vi "(C2K_ADC)_Config_Sweeps.vi"(8 "Error In":errorcluster, 10 "Parameter":T2, 11 "Front Panel Pop up":bool=TRUE) -> (0 "Error Out":errorcluster, 1 "VDDA":dbl[](array[numeric]), 2 "VDD":dbl[](array[numeric]), 3 "Temp":dbl[](array[numeric]), 4 "Parameter Out":T2, 5 "VDDIO":dbl[](array[numeric]))   [LabVIEW 2019]
uses:
  (C2K_ADC)_Array_cell_En_Dis.ctl
  (C2K_ADC)_Parameter.ctl
  (C2K_ADC)_Global.vi
panel:
  in  "VDDIO":T1
  out "name":string
  in  "Cancel Button":bool
  in  "OK Button":bool
  in  "Load Config":bool
  in  "Save Config":bool
  in  "VDDA":T1
  in  "VDD":T1
  in  "Temp":T1
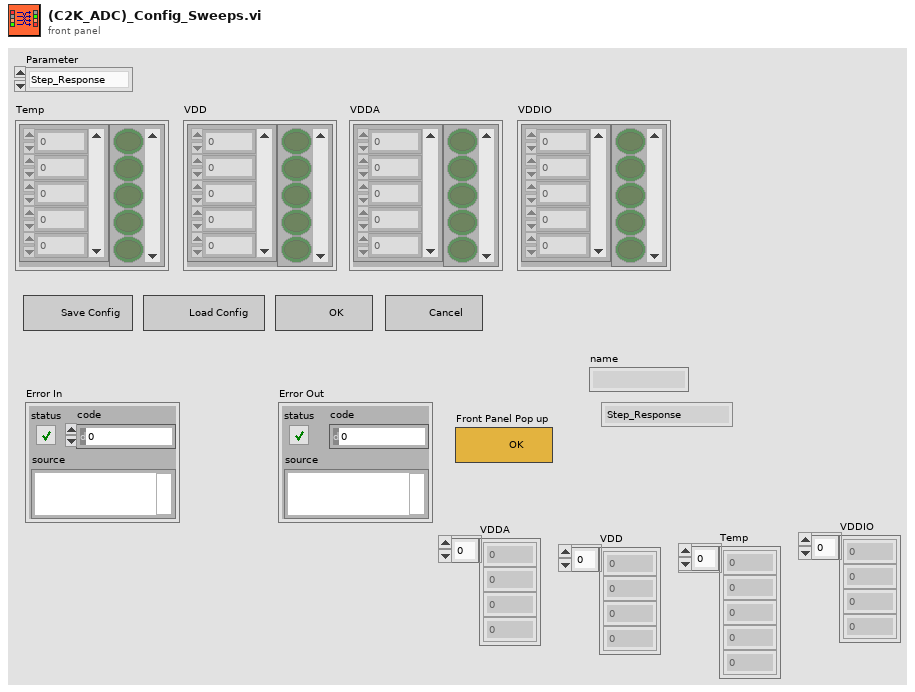
[diagram p1: front panel]
types:
  T1 = typedef "(C2K_ADC)_Array_cell_En_Dis.ctl" = cluster{"Array":dbl[], "Array 3":bool[]}
  T2 = typedef "(C2K_ADC)_Parameter.ctl" = enum16{"Step_Response"}
  T3 = enum32{"Invalid", "Standard", "Closed", "Hidden", "Minimized", "Maximized"}
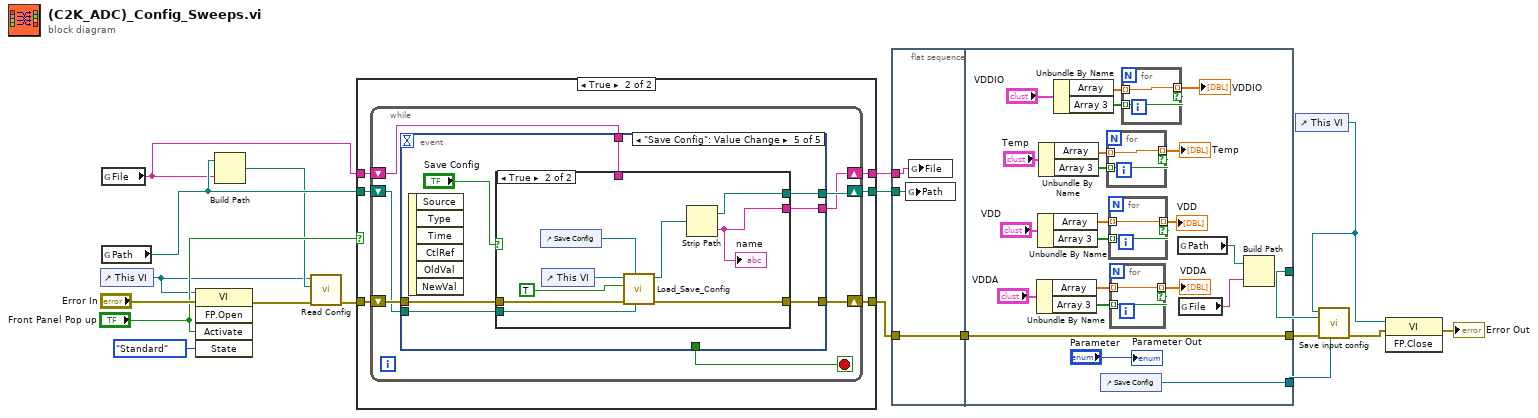
[diagram p0: block diagram]
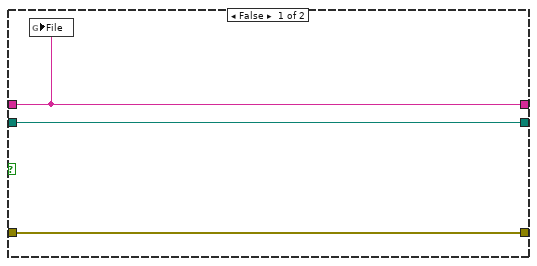
[diagram p2: hidden frame]
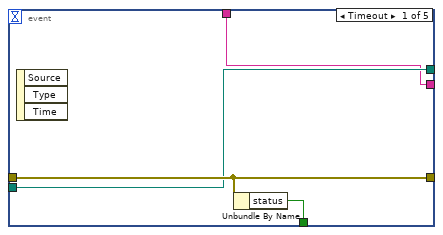
[diagram p3: hidden frame]
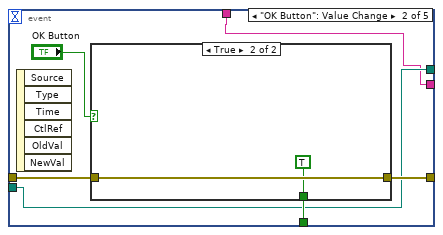
[diagram p4: hidden frame]
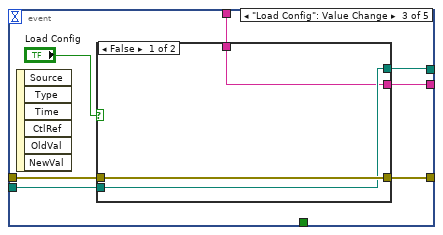
[diagram p6: hidden frame]
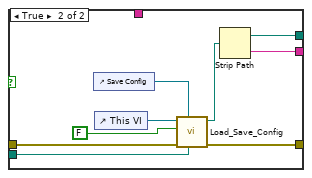
[diagram p7: hidden frame]
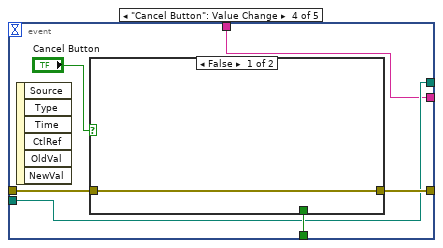
[diagram p8: hidden frame]
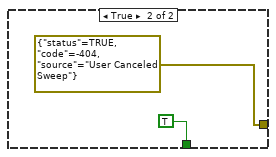
[diagram p9: hidden frame]
diagram:
  n1 = control-ref of="This VI"() -> (w9:refnum<vi>)
  n2 = global read "(C2K_ADC)_Global.vi" "File"() -> (w8:string)
  n3 = global read "(C2K_ADC)_Global.vi" "Path"() -> (w14:path)
  n4 = invoke class="VI" method="FP.Open"(reference=w9, error in="Error In", "Activate"="Front Panel Pop up", "State"=T3."Standard") -> (error out=w12:errorcluster)  [unwired: 1 in, 4 out]
  n5 = Build Path(base path=w14, name or relative path=w8) -> (appended path=w10:path)
  n6 = call <userlib>:"Read Config.vi"("error in"=w12, "file (use dialog)"=w10, "VI Reference"=w9) -> ("error out"=w11:errorcluster)  [unwired: 8 in]
  n7 = case shown="True" "Front Panel Pop up" {
    tunnel: [w22 w28] -> w19
    tunnel: [w21 w27] -> w18
    tunnel: w14 -> [w22 w26]
    tunnel: w11 -> [w21 w25]
    tunnel: w8 -> [w20 w23]
    tunnel: [w20 w24] -> w1
    frame False {
      n8 = global write "(C2K_ADC)_Global.vi" "File"(w20) -> ()
    }
    frame True {
      n9 = while {
        shift-right: [w34] -> w27
        shift-left: w25 -> [w35]
        shift-right: [w31] -> w28
        shift-left: w26 -> [w32]
        shift-right: [w30] -> w24
        shift-left: w23 -> [w29]
        stop <- w33 stop-if-true
        n10 = event shown="[4] \"Save Config\": Value Change" {
          selector: _ -> [_ _ _ _ _]
          dyn-events: _ -> [_ _ _ _ _]
          timeout: _ -> [_ _ _ _ _]
          tunnel: w35 -> [w39 w43 w54 w71 w82]
          tunnel: [w39 w44 w53 w70 w81] -> w34
          tunnel: [w38 w42 _ w72 _] -> w33
          tunnel: w32 -> [w37 w41 w52 w69 w80]
          tunnel: [w37 w41 w51 w69 w79] -> w31
          tunnel: [w36 w40 w50 w68 w78] -> w30
          tunnel: w29 -> [w36 w40 w49 w68 w77]
          event Timeout {
            n11 = event-data() -> ()  [unwired: 1 in, 3 out]
            n12 = Unbundle By Name(w39) -> ("status"=w38:bool)
          }
          event "OK Button": Value Change {
            n13 = event-data() -> ()  [unwired: 1 in, 6 out]
            n14 = case shown="True" "OK Button" {
              tunnel: [w46 w48] -> w44
              tunnel: w43 -> [w46 w48]
              tunnel: [_ TRUE] -> w42
              frame False {
              }
              frame True {
              }
            }
          }
          event "Load Config": Value Change {
            n15 = event-data() -> ()  [unwired: 1 in, 6 out]
            n16 = case shown="False" "Load Config" {
              tunnel: w54 -> [w58 w64]
              tunnel: [w58 w63] -> w53
              tunnel: w52 -> [w57 w62]
              tunnel: [w57 w60] -> w51
              tunnel: [w56 w59] -> w50
              tunnel: w49 -> [w56 _]
              frame False {
              }
              frame True {
                n17 = control-ref of="Save Config"() -> (w65:refnum<vi>)
                n18 = control-ref of="This VI"() -> (w66:refnum<vi>)
                n19 = call <userlib>:"Load_Save_Config.vi"("start path"=w62, "Save CTRL Reference"=w65, "error in (no error)"=w64, "Load /Save"=FALSE, "VI Reference"=w66) -> ("error out"=w63:errorcluster, "selected path"=w61:path)  [unwired: 5 in]
                n20 = Strip Path(path=w61) -> (stripped path=w60:path, name=w59:string)
              }
            }
          }
          event "Cancel Button": Value Change {
            n21 = event-data() -> ()  [unwired: 1 in, 6 out]
            n22 = case shown="False" "Cancel Button" {
              tunnel: [_ TRUE] -> w72
              tunnel: w71 -> [w74 _]
              tunnel: [w74 errorcluster {"status"=TRUE, "code"=-404, "source"="User Canceled Sweep"} ("error constant")] -> w70
              frame False {
              }
              frame True {
              }
            }
          }
          event "Save Config": Value Change {
            n23 = event-data() -> ()  [unwired: 1 in, 6 out]
            n24 = case shown="True" "Save Config" {
              tunnel: w82 -> [w86 w95]
              tunnel: [w86 w91] -> w81
              tunnel: w80 -> [w85 w90]
              tunnel: [w85 w88] -> w79
              tunnel: [w84 w87] -> w78
              tunnel: w77 -> [w84 _]
              frame False {
              }
              frame True {
                n25 = control-ref of="Save Config"() -> (w92:refnum<vi>)
                n26 = control-ref of="This VI"() -> (w93:refnum<vi>)
                n27 = call <userlib>:"Load_Save_Config.vi"("start path"=w90, "Save CTRL Reference"=w92, "error in (no error)"=w95, "Load /Save"=TRUE, "VI Reference"=w93) -> ("error out"=w91:errorcluster, "selected path"=w89:path)  [unwired: 5 in]
                n28 = Strip Path(path=w89) -> (stripped path=w88:path, name=w87:string)
                "name" <- w87
              }
            }
          }
        }
      }
    }
  }
  n29 = flat-sequence {
    tunnel: w19 -> [w97]
    tunnel: w18 -> [w98]
    tunnel: [w98] -> w2
    tunnel: w1 -> [w96]
    tunnel: [w108] -> w6
    tunnel: [w106] -> w5
    tunnel: [w103] -> w4
    tunnel: w2 -> [w108]
    frame #0 {
      n30 = global write "(C2K_ADC)_Global.vi" "Path"(w97) -> ()
      n31 = global write "(C2K_ADC)_Global.vi" "File"(w96) -> ()
    }
    frame #1 {
      n32 = Unbundle By Name("VDDA") -> ("Array"=w117:dbl[], "Array 3"=w116:bool[])
      n33 = Unbundle By Name("VDD") -> ("Array"=w114:dbl[], "Array 3"=w115:bool[])
      n34 = Unbundle By Name("Temp") -> ("Array"=w113:dbl[], "Array 3"=w112:bool[])
      n35 = Unbundle By Name("VDDIO") -> ("Array"=w101:dbl[], "Array 3"=w102:bool[])
      n36 = control-ref of="Save Config"() -> (w106:refnum<vi>)
      n37 = for {
        tunnel: w113 -> [w128] mode=indexing
        tunnel: w112 -> [w127] mode=indexing
        tunnel: [w128] -> w111 mode=indexing if=w127
      }
      "Temp" <- w111
      n38 = for {
        tunnel: w115 -> [w125] mode=indexing
        tunnel: w114 -> [w126] mode=indexing
        tunnel: [w126] -> w110 mode=indexing if=w125
      }
      "VDD" <- w110
      n39 = for {
        tunnel: w117 -> [w124] mode=indexing
        tunnel: w116 -> [w123] mode=indexing
        tunnel: [w124] -> w109 mode=indexing if=w123
      }
      "VDDA" <- w109
      n40 = for {
        tunnel: w101 -> [w122] mode=indexing
        tunnel: w102 -> [w121] mode=indexing
        tunnel: [w122] -> w99 mode=indexing if=w121
      }
      "VDDIO" <- w99
      n41 = global read "(C2K_ADC)_Global.vi" "Path"() -> (w105:path)
      n42 = global read "(C2K_ADC)_Global.vi" "File"() -> (w104:string)
      n43 = Build Path(base path=w105, name or relative path=w104) -> (appended path=w103:path)
      "Parameter Out" <- "Parameter"
    }
  }
  n44 = control-ref of="This VI"() -> (w7:refnum<vi>)
  n45 = call <userlib>:"Save input config.vi"("CTRL Reference"=w5, "error in (no error)"=w6, "Config File"=w4, "VI Reference"=w7) -> ("error out"=w3:errorcluster)  [unwired: 7 in]
  n46 = invoke class="VI" method="FP.Close"(reference=w7, error in=w3) -> (error out=→"Error Out":errorcluster)  [unwired: 1 in, 2 out]
